vi "WebSocket Write.vi"(6 "Mask payload?":bool, 8 "error in":errorcluster, 9 "timeout ms (5000)":i32=5000, 10 "Data":string, 11 "WebSocket Connection in":refnum<k5>) -> (0 "error out":errorcluster, 3 "WebSocket Connection out":refnum<k5>)   [LabVIEW 2018]
doc: "Sends a WebSocket message to the client. Messages sent from the client must be masked but it is optional for the server.\nWebSockets API 1.3.0.13\nSam Sharp - Intelligent Energy\nCopyright (c) 2015, Intelligent Energy"
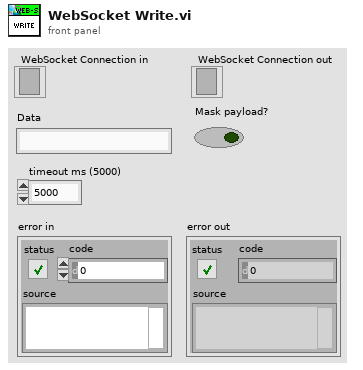
[diagram p1: front panel]
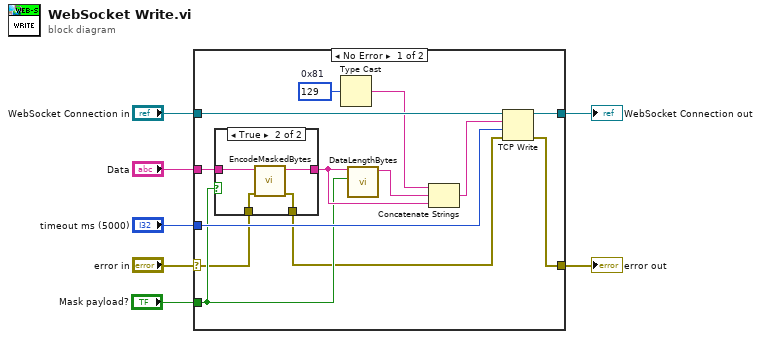
[diagram p0: block diagram]
diagram:
  n1 = case shown="No Error" "error in" {
    selector: "error in" -> [w9 w28]
    tunnel: [w18 w28] -> w6
    tunnel: [w20 w27] -> w4
    tunnel: "WebSocket Connection in" -> [w19 w27]
    tunnel: "Data" -> [w12 _]
    tunnel: "timeout ms (5000)" -> [w13 _]
    tunnel: "Mask payload?" -> [w10 _]
    frame No Error {
      w17 = u8 129  # 0x81
      n2 = case shown="True" w10 {
        tunnel: w12 -> [w22 w26]
        tunnel: [w22 w25] -> w11
        tunnel: w9 -> [w21 w24]
        tunnel: [w21 w23] -> w8
        frame False {
        }
        frame True {
          n3 = call "EncodeMaskedBytes.vi"("error in (no error)"=w24, "Raw Data"=w26) -> ("error out"=w23:errorcluster, "Encoded Data"=w25:string)  [unwired: 8 in]
        }
      }
      n4 = Type Cast(x=w17) -> (*(type *) &x=w15:string)  [unwired: 1 in]
      n5 = call "DataLengthBytes.vi"("Is masked?"=w10, "Data"=w11) -> ("Length Bytes"=w16:string)  [unwired: 9 in]
      n6 = Concatenate Strings(w15, w16, w11) -> (w14:string)
      n7 = TCP Write(connection ID=w19, data in=w14, error in (no error)=w8, 9:w13) -> (connection ID out=w20:refnum<k5>, error out=w18:errorcluster)  [unwired: 1 out]
    }
    frame Error {
    }
  }
  "WebSocket Connection out" <- w4
  "error out" <- w6
